vi "do_waveform_lite.vi"() -> ()   [LabVIEW 2020]
uses:
  <vilib>/Waveform/DWDTOps.llb/DWDT Analog to Digital.vi
panel:
  out "数字波形图":digitalwaveform(graph)={"t0"=timestamp(0 s since 1904-01-01), "dt"=1e-05, "Y"={"transitions"=[0, 1, 2, 3, 4, 5], "data"=[[0, 0, 0, 0], [0, 1, 0, 1], [1, 0, 1, 0], [0, 0, 0, 1], [1, 0, 0, 1], [0, 0, 0, 0]]}}
  in  "Value":u32[](array[numeric])=[8, 5, 10, 1, 9, 0] format="%04b"
  in  "DoCycle":u32=1
  out "error out":errorcluster caption="错误输出"
  in  "SamplePeriod(ns)":u32=10000
  in  "DevIndex":i32
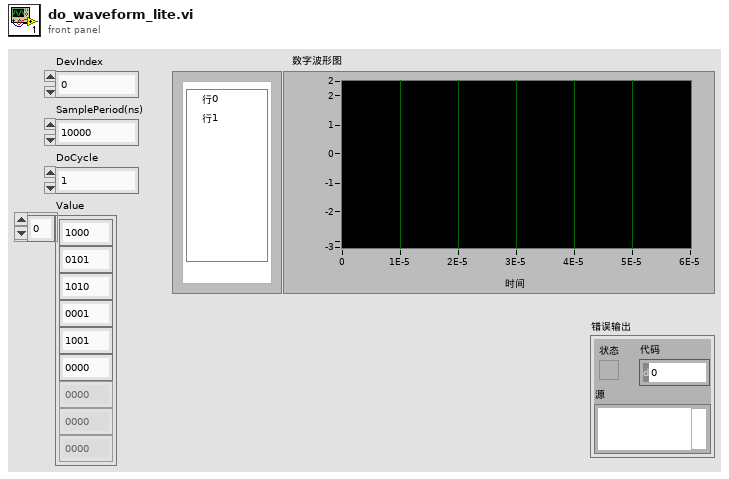
[diagram p1: front panel]
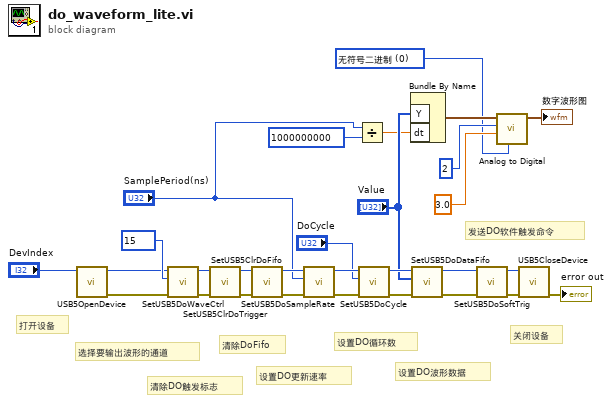
[diagram p0: block diagram]
diagram:
  w10 = u16 0 items=["无符号二进制", "二进制偏移量", "二进制补码"] ("data format (offset binary)")
  # "关闭设备"
  # "发送DO软件触发命令"
  # "设置DO波形数据"
  # "设置DO循环数"
  # "设置DO更新速率"
  # "清除DoFifo"
  # "清除DO触发标志"
  # "选择要输出波形的通道"
  # "打开设备"
  n1 = call "USB5OpenDevice.vi"("DevIndex"="DevIndex") -> ("error out"=w2:errorcluster, "DevIndex Out"=w3:i32)  [unwired: 9 in]
  n2 = call "SetUSB5DoWaveCtrl.vi"("错误输入（无错误）"=w2, "Chan"=u32 15, "DevIndex"=w3) -> ("错误输出"=w5:errorcluster, "DevIndex Out"=w6:i32)  [unwired: 7 in]
  n3 = call "SetUSB5ClrDoTrigger.vi"("错误输入（无错误）"=w5, "DevIndex"=w6) -> ("错误输出"=w26:errorcluster, "DevIndex Out"=w27:i32)  [unwired: 8 in]
  n4 = call "SetUSB5ClrDoFifo.vi"("错误输入（无错误）"=w26, "DevIndex"=w27) -> ("错误输出"=w24:errorcluster, "DevIndex Out"=w25:i32)  [unwired: 8 in]
  n5 = call "SetUSB5DoSampleRate.vi"("错误输入（无错误）"=w24, "SamplePeriod(ns)"="SamplePeriod(ns)", "DevIndex"=w25) -> ("错误输出"=w22:errorcluster, "DevIndex Out"=w23:i32)  [unwired: 7 in]
  n6 = Divide(x="SamplePeriod(ns)", y=u32 1000000000) -> (x/y=w7:dbl)
  n7 = call "SetUSB5DoCycle.vi"("错误输入（无错误）"=w22, "DoCycle"="DoCycle", "DevIndex"=w23) -> ("错误输出"=w19:errorcluster, "DevIndex Out"=w20:i32)  [unwired: 7 in]
  n8 = Bundle By Name ("创建波形")("Y"="Value", "dt"=w7) -> (w13:waveform(u32))  [unwired: 1 in]
  n9 = call "SetUSB5DoDataFifo.vi"("错误输入（无错误）"=w19, "Value"="Value", "DevIndex"=w20) -> ("错误输出"=w17:errorcluster, "DevIndex Out"=w18:i32)  [unwired: 7 in]
  n10 = call "SetUSB5DoSoftTrig.vi"("错误输入（无错误）"=w17, "DevIndex"=w18) -> ("错误输出"=w15:errorcluster, "DevIndex Out"=w16:i32)  [unwired: 8 in]
  n11 = call-poly <vilib>:"Analog to Digital.vi"("data format (offset binary)"=w10, "full-scale range (pk-pk)"=3.0, "resolution (16 bit)"=2, "analog waveform"=w13) -> ("digital waveform"=→"数字波形图":digitalwaveform)  [unwired: 4 in, 3 out]
  n12 = call "USB5CloseDevice.vi"("错误输入（无错误）"=w15, "DevIndex"=w16) -> ("error out"=→"error out":errorcluster)  [unwired: 8 in, 1 out]
